vi "GFGfpRefGet.vi"(7 "GFG Refnum (use when calling from external project)":refnum<vi>, 8 "error in (no error)":errorcluster, 11 "Variable Name in":string) -> (0 "error out":errorcluster, 3 "output cluster":T1)   [LabVIEW 2012, in "GFG library.lvlib"]
uses:
  GFG library.lvlib
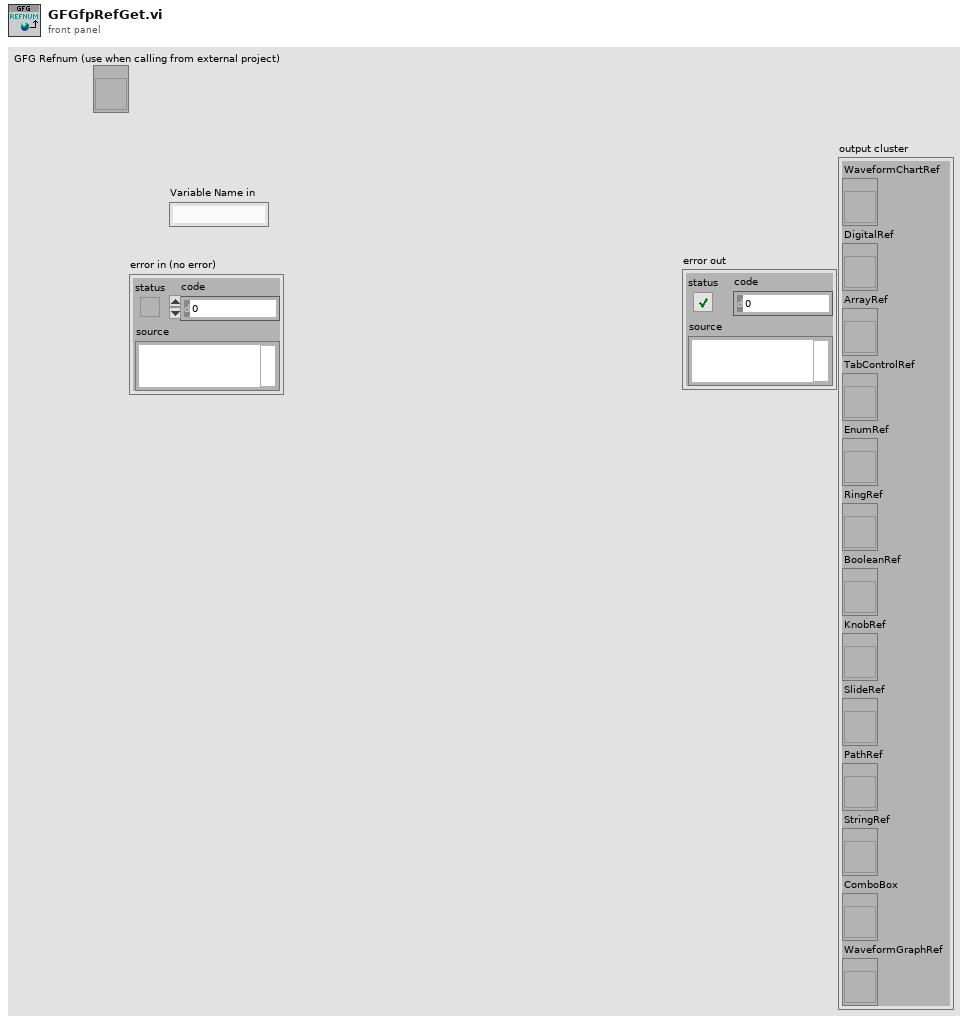
[diagram p1: front panel]
types:
  T1 = cluster{"WaveformChartRef":refnum<vi>, "DigitalRef":refnum<vi>, "ArrayRef":refnum<vi>, "TabControlRef":refnum<vi>, "EnumRef":refnum<vi>, "RingRef":refnum<vi>, "BooleanRef":refnum<vi>, "KnobRef":refnum<vi>, "SlideRef":refnum<vi>, "PathRef":refnum<vi>, "StringRef":refnum<vi>, "ComboBox":refnum<vi>, "WaveformGraphRef":refnum<vi>}
  T2 = typedef "VariantType.lvlib/Type.ctl" = enum8{"Invalid Type", "Void", "I8", "I16", "I32", "I64", "U8", "U16", "U32", "U64", "Single Float", "Double Float", "Extended Float", "Single Complex", "Double Complex", "Extended Complex", "Enum U8", "Enum U16", "Enum U32", "Enum U64", "Single Float With Unit", "Double Float With Unit", "Extended Float With Unit", "Single Complex with Unit", "Double Complex with Unit", "Extended Complex with Unit", "Boolean", "String", "Path", "Picture", "Tag", "Array", "Cluster", "Variant", "LV Variant", "Waveform", "Timestamp", "Digital Waveform", "Digital Data", "ExpressData", "Refnum", "External Data", "VI", "Poly VI", "LabVIEW Class Instance", "Fixed Point"}
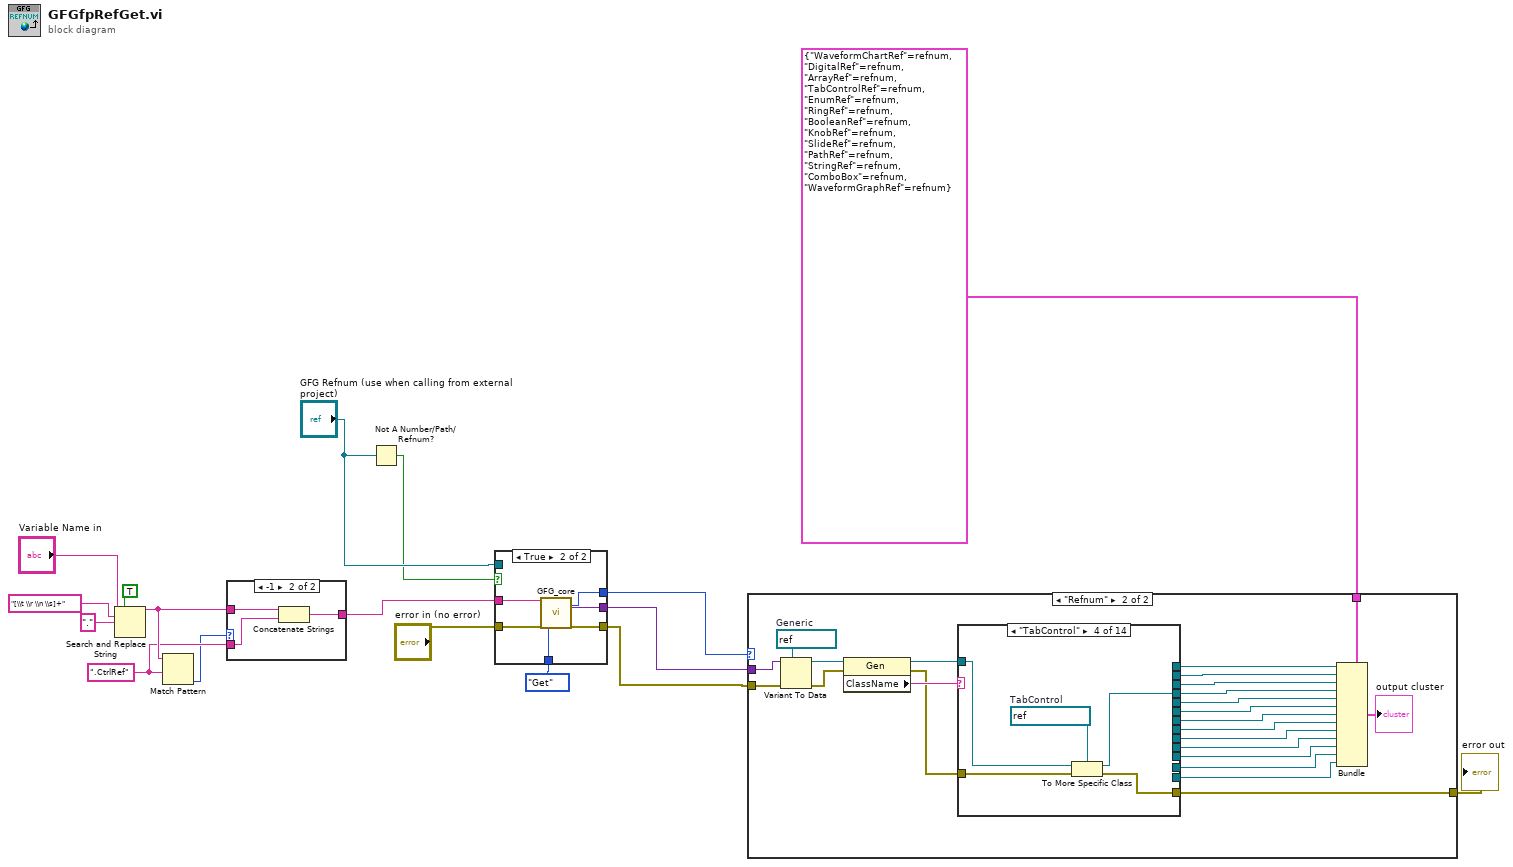
[diagram p0: block diagram]
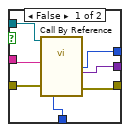
[diagram p2: hidden frame]
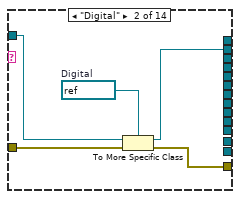
[diagram p6: hidden frame]
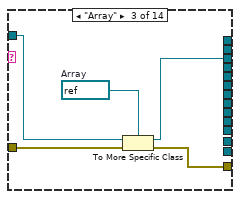
[diagram p7: hidden frame]
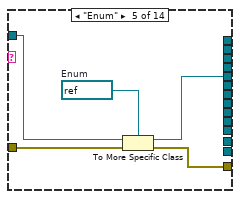
[diagram p8: hidden frame]
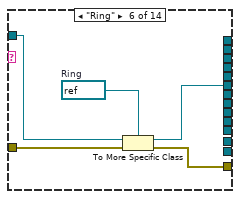
[diagram p9: hidden frame]
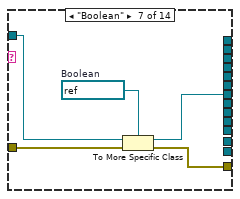
[diagram p10: hidden frame]
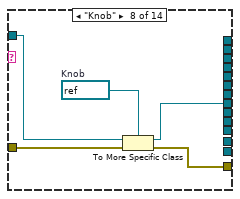
[diagram p11: hidden frame]
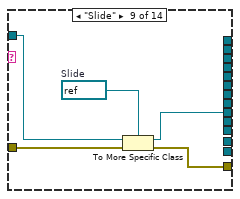
[diagram p12: hidden frame]
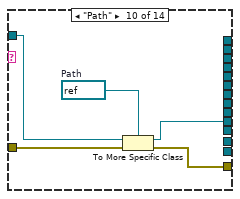
[diagram p13: hidden frame]
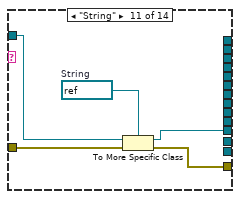
[diagram p14: hidden frame]
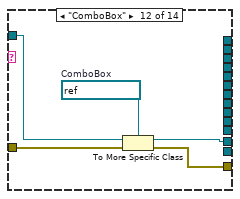
[diagram p15: hidden frame]
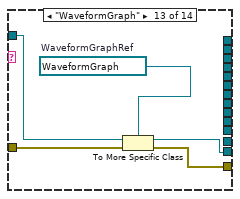
[diagram p16: hidden frame]
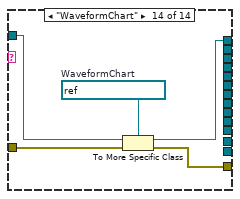
[diagram p17: hidden frame]
diagram:
  w11 = ".CtrlRef" ("string")
  n1 = Search and Replace String(replace all?=TRUE ("replace all? (F)"), input string="Variable Name in", search string="[\\t \\r \\n \\s]+", replace string="." ("replace string (\"\")")) -> (result string=w12:string)  [unwired: 4 in, 3 out]
  n2 = Match Pattern(string=w12, regular expression=w11) -> (offset past match=w10:i32)  [unwired: 1 in, 3 out]
  n3 = case shown="-1" w10 {
    tunnel: [w18 w21] -> w5
    tunnel: w12 -> [w18 w20]
    tunnel: w11 -> [_ w19]
    frame 0, Default {
    }
    frame -1 {
      n4 = Concatenate Strings(w20, w19) -> (w21:string)
    }
  }
  n5 = Not A Number/Path/Refnum?(number/path/refnum="GFG Refnum (use when calling from external project)") -> (NaN/Path/Refnum?=w6:bool)
  n6 = case shown="True" w6 {
    tunnel: enum16{"Init", "Set", "Get"}."Get" ("Action") -> [w23 w34]
    tunnel: w5 -> [w24 w33]
    tunnel: "error in (no error)" -> [w28 w32]
    tunnel: [w27 w31] -> w3
    tunnel: [w25 w30] -> w2
    tunnel: [w26 w29] -> w1
    tunnel: "GFG Refnum (use when calling from external project)" -> [w22 _]
    frame False {
      n7 = call-by-ref "?"(reference=w22, "Variable Name in"=w24, "error in (no error)"=w28, "Action"=w23) -> ("Data Type Out"=w25:T2, "Variant Out"=w26:variant, "error out"=w27:errorcluster)  [unwired: 11 in, 6 out]
    }
    frame True {
      n8 = call "GFG_core.vi"("Variable Name in"=w33, "error in (no error)"=w32, "Action"=w34) -> ("Data Type Out"=w30:T2, "Variant Out"=w29:variant, "error out"=w31:errorcluster)  [unwired: 10 in, 4 out]
    }
  }
  n9 = case shown="\"Refnum\"" w2 {
    tunnel: w1 -> [_ w59]
    tunnel: w3 -> [w35 w58]
    tunnel: [w35 w53] -> w17
    tunnel: T1 {"WaveformChartRef"=refnum, "DigitalRef"=refnum, "ArrayRef"=refnum, "TabControlRef"=refnum, "EnumRef"=refnum, "RingRef"=refnum, "BooleanRef"=refnum, "KnobRef"=refnum, "SlideRef"=refnum, "PathRef"=refnum, "StringRef"=refnum, "ComboBox"=refnum, "WaveformGraphRef"=refnum} ("output cluster") -> [_ w38]
    frame Default {
    }
    frame "Refnum" {
      w57 = refnum<vi> refnum  # Generic
      n10 = Variant To Data(error in=w58, type=w57, Variant=w59) -> (data=w56:refnum<vi>, error out=w41:errorcluster)
      n11 = property class="Gen"(reference=w56, error in=w41) -> (reference out=w54:refnum<vi>, error out=w40:errorcluster, "ClassName"=w55:string)
      n12 = case shown="\"TabControl\"" w55 {
        tunnel: w54 -> [_ w64 w69 w74 w79 w84 w89 w94 w99 w104 w109 w114 w120 w124]
        tunnel: [_ _ _ _ _ _ _ _ _ _ _ _ _ w123] -> w52
        tunnel: [_ w63 _ _ _ _ _ _ _ _ _ _ _ _] -> w51
        tunnel: w40 -> [w60 w62 w67 w72 w76 w82 w86 w91 w96 w101 w106 w112 w118 w121]
        tunnel: [w60 w61 w66 w71 w77 w81 w87 w92 w97 w102 w107 w113 w119 w122] -> w53
        tunnel: [_ _ w68 _ _ _ _ _ _ _ _ _ _ _] -> w50
        tunnel: [_ _ _ w73 _ _ _ _ _ _ _ _ _ _] -> w49
        tunnel: [_ _ _ _ w78 _ _ _ _ _ _ _ _ _] -> w48
        tunnel: [_ _ _ _ _ w83 _ _ _ _ _ _ _ _] -> w47
        tunnel: [_ _ _ _ _ _ w88 _ _ _ _ _ _ _] -> w46
        tunnel: [_ _ _ _ _ _ _ w93 _ _ _ _ _ _] -> w45
        tunnel: [_ _ _ _ _ _ _ _ w98 _ _ _ _ _] -> w44
        tunnel: [_ _ _ _ _ _ _ _ _ w103 _ _ _ _] -> w43
        tunnel: [_ _ _ _ _ _ _ _ _ _ w108 _ _ _] -> w42
        tunnel: [_ _ _ _ _ _ _ _ _ _ _ w111 _ _] -> w39
        tunnel: [_ _ _ _ _ _ _ _ _ _ _ _ w117 _] -> w37
        frame "False", Default {
        }
        frame "Digital" {
          w65 = refnum<vi> refnum  # Digital
          n13 = To More Specific Class(target class=w65, reference=w64, error in=w62) -> (specific class reference=w63:refnum<vi>, error out=w61:errorcluster)
        }
        frame "Array" {
          w70 = refnum<vi> refnum  # Array
          n14 = To More Specific Class(target class=w70, reference=w69, error in=w67) -> (specific class reference=w68:refnum<vi>, error out=w66:errorcluster)
        }
        frame "TabControl" {
          w75 = refnum<vi> refnum  # TabControl
          n15 = To More Specific Class(target class=w75, reference=w74, error in=w72) -> (specific class reference=w73:refnum<vi>, error out=w71:errorcluster)
        }
        frame "Enum" {
          w80 = refnum<vi> refnum  # Enum
          n16 = To More Specific Class(target class=w80, reference=w79, error in=w76) -> (specific class reference=w78:refnum<vi>, error out=w77:errorcluster)
        }
        frame "Ring" {
          w85 = refnum<vi> refnum  # Ring
          n17 = To More Specific Class(target class=w85, reference=w84, error in=w82) -> (specific class reference=w83:refnum<vi>, error out=w81:errorcluster)
        }
        frame "Boolean" {
          w90 = refnum<vi> refnum  # Boolean
          n18 = To More Specific Class(target class=w90, reference=w89, error in=w86) -> (specific class reference=w88:refnum<vi>, error out=w87:errorcluster)
        }
        frame "Knob" {
          w95 = refnum<vi> refnum  # Knob
          n19 = To More Specific Class(target class=w95, reference=w94, error in=w91) -> (specific class reference=w93:refnum<vi>, error out=w92:errorcluster)
        }
        frame "Slide" {
          w100 = refnum<vi> refnum  # Slide
          n20 = To More Specific Class(target class=w100, reference=w99, error in=w96) -> (specific class reference=w98:refnum<vi>, error out=w97:errorcluster)
        }
        frame "Path" {
          w105 = refnum<vi> refnum  # Path
          n21 = To More Specific Class(target class=w105, reference=w104, error in=w101) -> (specific class reference=w103:refnum<vi>, error out=w102:errorcluster)
        }
        frame "String" {
          w110 = refnum<vi> refnum  # String
          n22 = To More Specific Class(target class=w110, reference=w109, error in=w106) -> (specific class reference=w108:refnum<vi>, error out=w107:errorcluster)
        }
        frame "ComboBox" {
          w115 = refnum<vi> refnum  # ComboBox
          n23 = To More Specific Class(target class=w115, reference=w114, error in=w112) -> (specific class reference=w111:refnum<vi>, error out=w113:errorcluster)
        }
        frame "WaveformGraph" {
          w116 = refnum<vi> refnum  # WaveformGraphRef
          n24 = To More Specific Class(target class=w116, reference=w120, error in=w118) -> (specific class reference=w117:refnum<vi>, error out=w119:errorcluster)
        }
        frame "WaveformChart" {
          w125 = refnum<vi> refnum  # WaveformChart
          n25 = To More Specific Class(target class=w125, reference=w124, error in=w121) -> (specific class reference=w123:refnum<vi>, error out=w122:errorcluster)
        }
      }
      n26 = Bundle(cluster=w38, "WaveformChartRef"=w52, "DigitalRef"=w51, "ArrayRef"=w50, "TabControlRef"=w49, "EnumRef"=w48, "RingRef"=w47, "BooleanRef"=w46, "KnobRef"=w45, "SlideRef"=w44, "PathRef"=w43, "StringRef"=w42, "ComboBox"=w39, "WaveformGraphRef"=w37) -> (→"output cluster":T1)
    }
  }
  "error out" <- w17
